vi "Shutdown.vi"(8 "error in (no error)":errorcluster, 11 "Laser_Oxxius in":refnum<class "Laser_Oxxius.lvclass">) -> (0 "error out":errorcluster, 3 "Laser_Oxxius out":refnum<class "Laser_Oxxius.lvclass">)   [LabVIEW 2020, in "Laser_Oxxius.lvlib" / "Laser_Oxxius.lvclass"]
uses:
  Laser_Oxxius.lvclass
  E:/Development/DevHardSoftware/MicroscopyFramework/Model/Hardware Layer/Real Hardware/Laser_Oxxius/Laser_Oxxius/Dependency/Oxxius_Boxx.dll
  Dependency/Oxxius_Boxx.dll
  Hardware Abstraction Layer/Component/Laser/Laser/Laser.lvclass
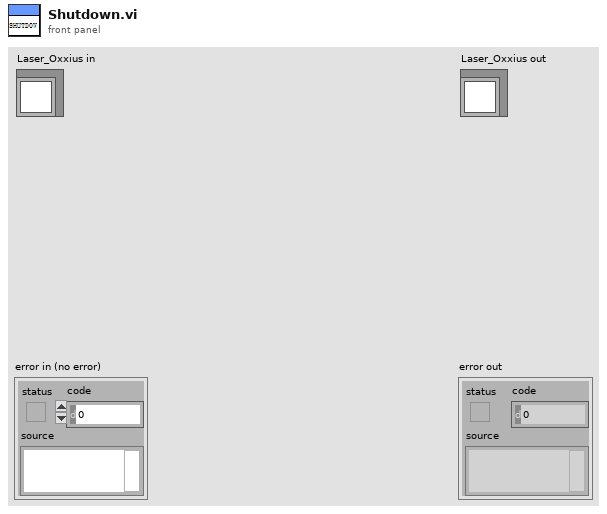
[diagram p1: front panel]
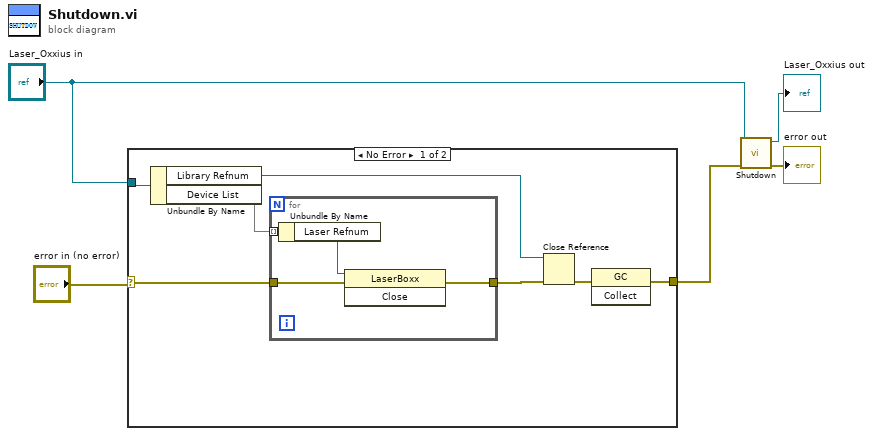
[diagram p0: block diagram]
diagram:
  n1 = case shown="No Error" "error in (no error)" {
    selector: "error in (no error)" -> [w10 w17]
    tunnel: [w6 w17] -> w1
    tunnel: "Laser_Oxxius in" -> [w12 _]
    frame No Error {
      n2 = Unbundle By Name(w12) -> ("Library Refnum"=w8:refnum<k24>, "Device List"=w11:map{string, refnum<k24>})
      n3 = for {
        tunnel: w11 -> [w16] mode=indexing
        tunnel: w10 -> [w14]
        tunnel: [w13] -> w9
        n4 = Unbundle By Name(w16) -> ("Laser Refnum"=w15:refnum<k24>)
        n5 = invoke class="LaserBoxx" method="Close"(reference=w15, error in=w14) -> (error out=w13:errorcluster)  [unwired: 1 in, 2 out]
      }
      n6 = Close Reference(reference=w8, error in (no error)=w9) -> (error out=w7:errorcluster)
      n7 = invoke class="GC" method="Collect"(error in=w7) -> (error out=w6:errorcluster)  [unwired: 2 in, 2 out]
    }
    frame Error {
    }
  }
  n8 = call-parent "Shutdown.vi"("error in (no error)"=w1, "GRMActor in"="Laser_Oxxius in") -> ("error out"=→"error out":errorcluster, "GRMActor out"=→"Laser_Oxxius out":refnum<class "Laser_Oxxius.lvclass">)  [unwired: 8 in]
